vi "create StringPayload.vi"(8 "error in (no error)":errorcluster, 10 "String":string, 11 "StringPayload in":refnum<class "StringPayload.lvclass">) -> (0 "error out":errorcluster, 3 "StringPayload out":refnum<class "StringPayload.lvclass">)   [LabVIEW 2019, in "StringPayload.lvclass"]
uses:
  StringPayload.lvclass
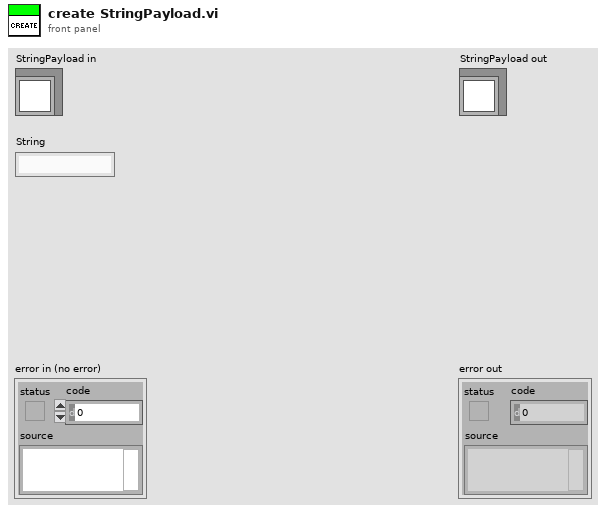
[diagram p1: front panel]
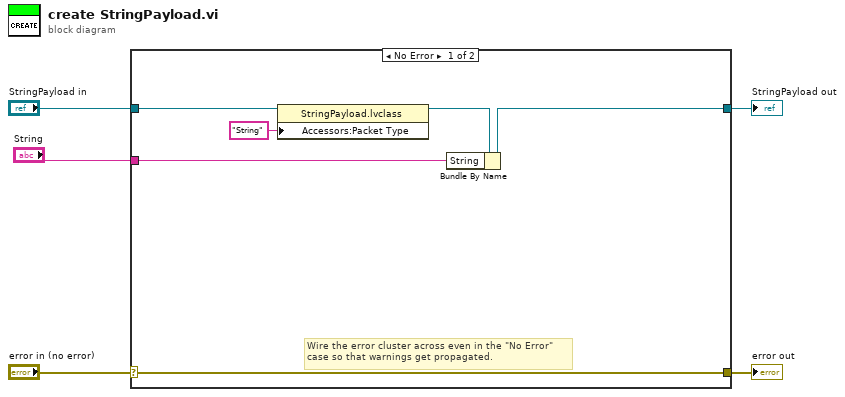
[diagram p0: block diagram]
diagram:
  n1 = case shown="No Error" "error in (no error)" {
    selector: "error in (no error)" -> [w10 w13]
    tunnel: [w10 w13] -> w4
    tunnel: [w9 w12] -> w2
    tunnel: "StringPayload in" -> [w11 w12]
    tunnel: "String" -> [w8 _]
    frame No Error {
      # "Wire the error cluster across even in the \"No Error\"\ncase so that warnings get propagated."
      n2 = property class="StringPayload.lvclass"(reference=w11, "Accessors:Packet Type"="String" ("Packet Type")) -> (reference out=w7:refnum<class "StringPayload.lvclass">)  [unwired: 1 in, 1 out]
      n3 = Bundle By Name(cluster=w7, "String"=w8) -> (w9:refnum<class "StringPayload.lvclass">)
    }
    frame Error {
    }
  }
  "error out" <- w4
  "StringPayload out" <- w2
